vi "udp receive from python.vi"() -> ()   [LabVIEW 2017]
uses:
  global variable.vi
panel:
  out "data out":T1
  in  "Stop":bool
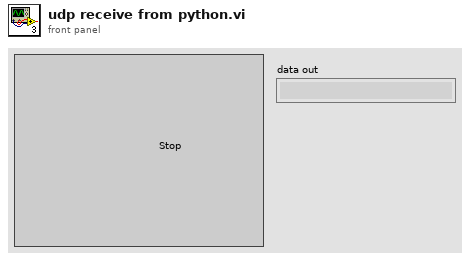
[diagram p1: front panel]
types:
  T1 = typedef "컨트롤 1.ctl" = string
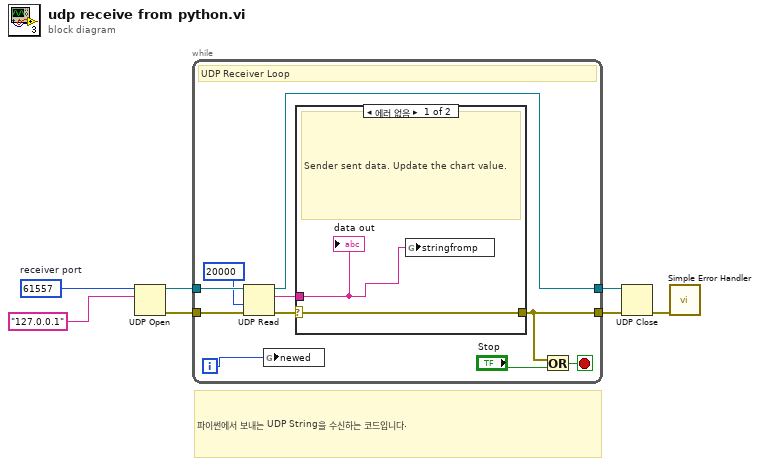
[diagram p0: block diagram]
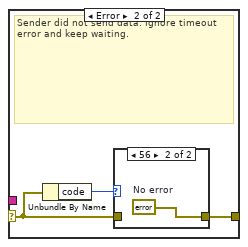
[diagram p2: hidden frame]
diagram:
  w2 = u16 61557  # receiver port
  # "파이썬에서 보내는 UDP String을 수신하는 코드입니다."
  n1 = UDP Open(10:"127.0.0.1" ("서비스 이름"), 11:w2) -> (port=w3:refnum<k16>, 0:w4:errorcluster)  [unwired: 3 in, 1 out]
  n2 = while {
    tunnel: w3 -> [w17]
    tunnel: [w9] -> w7
    tunnel: w4 -> [w14]
    tunnel: [w10] -> w5
    i -> [w8]
    stop <- w15 stop-if-true
    # "UDP Receiver Loop"
    n3 = UDP Read(connection ID=w17, timeout ms (25000)=20000, 8:w14) -> (data out=w12:string, error out=w11:errorcluster, 3:w9:refnum<k16>)  [unwired: 3 out]
    n4 = global write "global variable.vi" "newed"(w8) -> ()
    n5 = case shown="에러 없음" w11 {
      selector: w11 -> [w19 w21]
      tunnel: w12 -> [w18 _]
      tunnel: [w19 w20] -> w10
      frame No Error {
        # "Sender sent data. Update the chart value."
        n6 = global write "global variable.vi" "stringfromp"(w18) -> ()
        "data out" <- w18
      }
      frame Error {
        # "Sender did not send data. Ignore timeout error and keep waiting."
        n7 = Unbundle By Name(w21) -> ("code"=w22:i32)
        n8 = case shown="56" w22 {
          tunnel: w21 -> [w23 _]
          tunnel: [w23 w24] -> w20
          frame Default {
          }
          frame 56 {
            w24 = errorcluster {"status"=FALSE, "code"=0, "source"=""}  # No error
          }
        }
      }
    }
    n9 = Or(x=w10, y="Stop") -> (x .or. y?=w15:bool)
  }
  n10 = UDP Close(connection ID=w7, 8:w5) -> (error out=w6:errorcluster)  [unwired: 1 out]
  n11 = call <vilib>:"Simple Error Handler.vi"("error in (no error)"=w6) -> ()  [unwired: 1 in, 8 out]
